vi "Binary counter (for generating possible msg signals)(SubVI).vi"(1 "k":dbl) -> (0 "msg words":i16[][](array[numeric]))   [LabVIEW 2014]
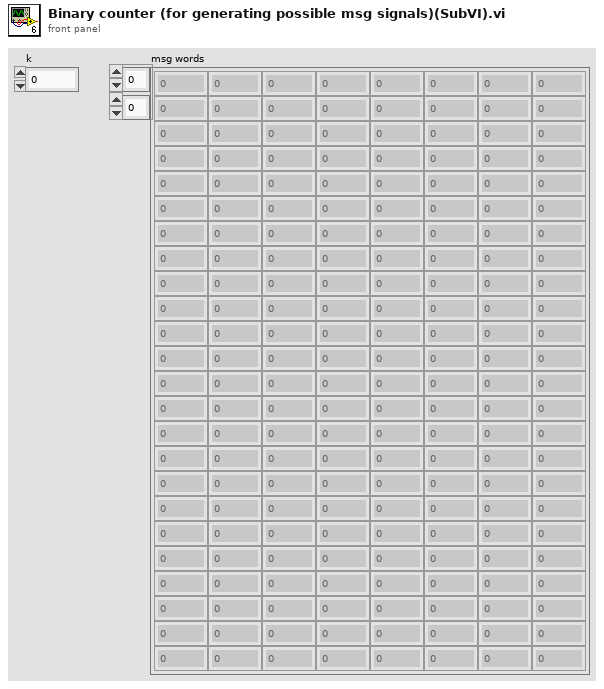
[diagram p1: front panel]
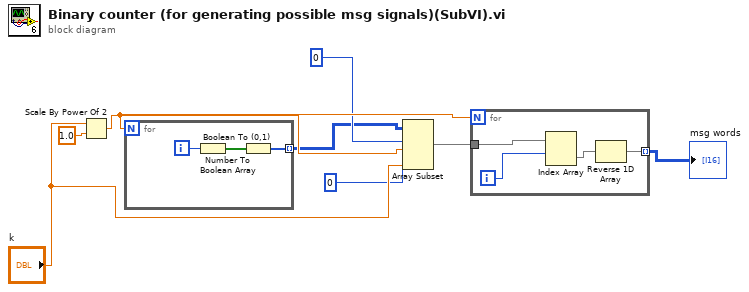
[diagram p0: block diagram]
diagram:
  n1 = Scale By Power Of 2(n="k", x=1.0) -> (x*2^n=w8:dbl)
  n2 = for {
    N: w8 -> [_]
    tunnel: [w9] -> w2 mode=indexing
    i -> [w10]
    n3 = Number To Boolean Array(number=w10) -> (Boolean array=w11:bool[])
    n4 = Boolean To (0,1)(Boolean=w11) -> (0, 1=w9:i16[])
  }
  n5 = Array Subset(array=w2, index (row)=0 ("index"), length (row)=w8, index (col)=0 ("index 2"), length (col)="k") -> (w5:i16[][])
  n6 = for {
    N: w8 -> [_]
    tunnel: w5 -> [w15]
    tunnel: [w12] -> w7 mode=indexing
    i -> [w13]
    n7 = Index Array(array=w15, index (row)=w13) -> (element=w14:i16[])  [unwired: 1 in]
    n8 = Reverse 1D Array(array=w14) -> (reversed array=w12:i16[])
  }
  "msg words" <- w7
